vi "Write Config to File.vi"(6 "Comment out unparsable lines":bool, 7 "Write even if no changes":bool, 8 "error in (no error)":errorcluster, 9 "Original Config":string="{}", 10 "New Config":string="{}", 11 "config file path":path) -> (0 "error out":errorcluster, 2 "<JSON>Config as Written":string, 4 "<JSON>As in file (before changes)":string)   [LabVIEW 2020, in "Config File.lvclass"]
doc: "Merges an Object into another JSON Object.\n\nMerging means that each item of the \"Object to merge\" is inserted into the other object. Insertion is at the root level unless a Path to a subObject is specified.\n\nExample: Merging {\"a\":1,\"b\":2} into {\"a\":3,\"c\":4} gives {\"a\":1,\"c\": 4,\"b\":2}\n\nNote that this merging is not recursive into subObjects."
uses:
  <vilib>/JDP Science/JSONtext/Config Files/Config File.lvclass
  <vilib>/JDP Science/JSONtext/support/Format Error.vi
  <vilib>/JDP Science/JSONtext/JSON type.vi
  <vilib>/Utility/error.llb/Error Cluster From Error Code.vi
  <vilib>/JDP Science/JSONtext/JSONtext.lvlib
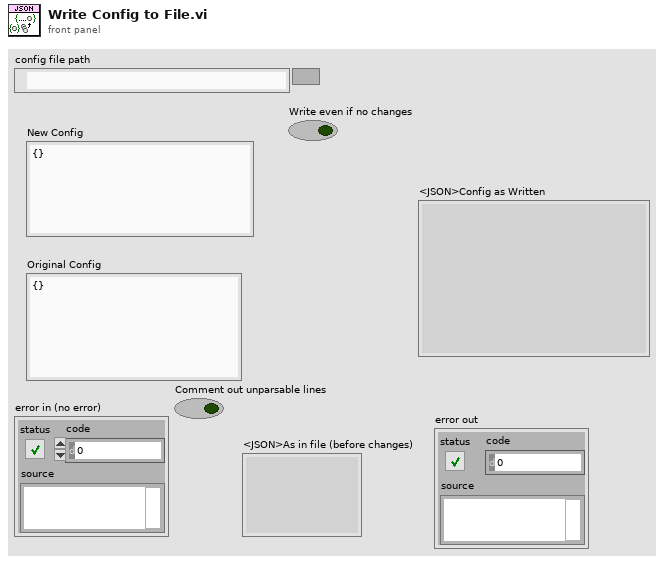
[diagram p1: front panel]
types:
  T1 = enum16{"deny read/write", "deny write-only", "deny none"}
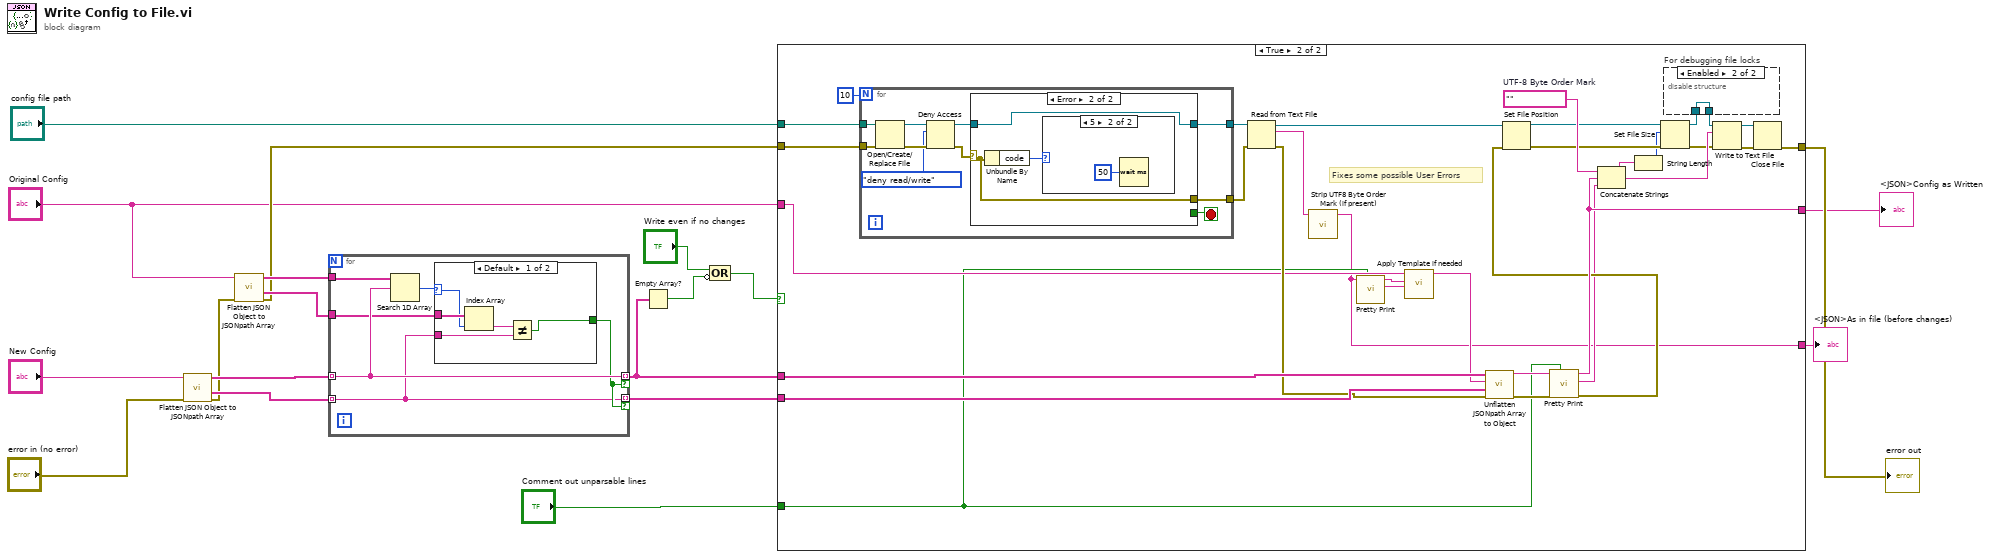
[diagram p0: block diagram]
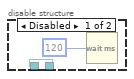
[diagram p3: hidden frame]
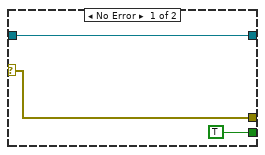
[diagram p4: hidden frame]
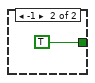
[diagram p6: hidden frame]
diagram:
  n1 = call <vilib>:"Flatten JSON Object to JSONpath Array.vi"("error in (no error)"="error in (no error)", "JSON"="New Config") -> ("error out"=w11:errorcluster, "<JSON>"=w15:string[], "$Paths"=w17:string[])  [unwired: 7 in]
  n2 = call <vilib>:"Flatten JSON Object to JSONpath Array.vi"("error in (no error)"=w11, "JSON"="Original Config") -> ("error out"=w10:errorcluster, "<JSON>"=w14:string[], "$Paths"=w16:string[])  [unwired: 7 in]
  n3 = for {
    tunnel: w17 -> [w23] mode=indexing
    tunnel: w16 -> [w25]
    tunnel: [w23] -> w8 mode=indexing if=w22
    tunnel: [w21] -> w13 mode=indexing if=w22
    tunnel: w15 -> [w21] mode=indexing
    tunnel: w14 -> [w20]
    n4 = Search 1D Array(1D array=w25, element=w23) -> (index of element=w24:i32)  [unwired: 1 in]
    n5 = case shown="Default" w24 {
      selector: w24 -> [w28 _]
      tunnel: [w26 TRUE] -> w22
      tunnel: w21 -> [w30 _]
      tunnel: w20 -> [w29 _]
      frame Default {
        n6 = Index Array(array=w29, index=w28) -> (element=w27:string)
        n7 = Not Equal?(x=w27, y=w30) -> (x != y?=w26:bool)
      }
      frame -1 {
      }
    }
  }
  n8 = Empty Array?(array=w8) -> (empty?=w4:bool)
  n9 = Compound Arithmetic op=OR("Write even if no changes", invert w4) -> (w3:bool)
  n10 = case shown="True" w3 {
    tunnel: "config file path" -> [_ w64]
    tunnel: w8 -> [_ w61]
    tunnel: w13 -> [_ w60]
    tunnel: w10 -> [w32 w59]
    tunnel: [w32 w55] -> w9
    tunnel: [_ w52] -> w7
    tunnel: "Original Config" -> [_ w45]
    tunnel: "Comment out unparsable lines" -> [_ w34]
    tunnel: [_ w33] -> w1
    frame False {
    }
    frame True {
      w49 = "﻿"  # UTF-8 Byte Order Mark
      # "Fixes some possible User Errors"
      n11 = for {
        N: 10 -> [_]
        tunnel: w64 -> [w77]
        tunnel: [w72] -> w63
        tunnel: w59 -> [w70]
        tunnel: [w69] -> w58
        stop <- w71 stop-if-true
        n12 = Open/Create/Replace File(file path (use dialog)=w77, error in=w70) -> (refnum out=w75:refnum<file>, error out=w76:errorcluster)  [unwired: 4 in, 1 out]
        n13 = Deny Access(4:w76, 6:T1."deny read/write" ("deny mode (0:deny read/write)"), 7:w75) -> (0:w74:errorcluster, 3:w73:refnum<file>)
        n14 = case shown="Error" w74 {
          selector: w74 -> [w78 w81]
          tunnel: w73 -> [w80 w82]
          tunnel: [w80 w82] -> w72
          tunnel: [TRUE _] -> w71
          tunnel: [w78 w81] -> w69
          frame No Error {
          }
          frame Error {
            n15 = Unbundle By Name(w81) -> ("code"=w83:i32)
            n16 = case shown="5" w83 {
              frame 0, Default {
              }
              frame 5 {
                n17 = Wait (ms)(milliseconds to wait=u32 50) -> ()  [unwired: 1 out]
              }
            }
          }
        }
      }
      n18 = Read from Text File(file (use dialog)=w63, error in=w58) -> (refnum out=w56:refnum<file>, text=w62:string, error out=w57:errorcluster)  [unwired: 2 in, 1 out]
      n19 = call <vilib>:"Strip UTF8 Byte Order Mark (if present).vi"("Text in"=w62) -> ("Possible Byte Order Mark Stripped"=w33:string)  [unwired: 9 in, 1 out]
      n20 = call <vilib>:"Pretty Print.vi"("Comment out unparsable lines"=w34, "JSON"=w33) -> ("Rest of Input String"=w47:string, "<JSON>"=w46:string)  [unwired: 7 in, 1 out]
      n21 = call <vilib>:"Apply Template if needed.vi"("Rest of Input String"=w47, "From File"=w46, "Template"=w45) -> ("<JSON>"=w48:string)  [unwired: 6 in, 2 out]
      n22 = call <vilib>:"Unflatten JSONpath Array to Object.vi"("error in (no error)"=w57, "JSON Items"=w60, "Initial JSON Object"=w48, "$Paths"=w61) -> ("error out"=w51:errorcluster, "<JSON>"=w53:string)  [unwired: 6 in]
      n23 = call <vilib>:"Pretty Print.vi"("Comment out unparsable lines"=w34, "error in (no error)"=w51, "JSON"=w53) -> ("error out"=w50:errorcluster, "Rest of Input String"=w44:string, "<JSON>"=w52:string)  [unwired: 6 in]
      n24 = Set File Position(refnum=w56, error in=w50) -> (refnum out=w40:refnum<file>, error out=w39:errorcluster)  [unwired: 2 in]
      n25 = Concatenate Strings(w49, w52, w44) -> (w41:string)
      n26 = String Length(string=w41) -> (length=w37:i32)
      n27 = Set File Size(4:w39, 6:w37, 7:w40) -> (0:w38:errorcluster, 3:w36:refnum<file>)
      n28 = disable-structure "For debugging file locks" shown="Enabled" {
        disable-tunnel: w36 -> [w65 w67]
        disable-tunnel: [w65 w67] -> w35
        frame Disabled {
          n29 = Wait (ms)(milliseconds to wait=u32 120) -> ()  [unwired: 1 out]
        }
        frame Enabled {
        }
      }
      n30 = Write to Text File(file (use dialog)=w35, text=w41, error in=w38) -> (refnum out=w43:refnum<file>, error out=w42:errorcluster)  [unwired: 1 in, 1 out]
      n31 = Close File(refnum=w43, error in=w42) -> (error out=w55:errorcluster)  [unwired: 1 out]
    }
  }
  "error out" <- w9
  "<JSON>Config as Written" <- w7
  "<JSON>As in file (before changes)" <- w1
